vi "Start over Tracking v2.vi"(3 "error in (no error)":errorcluster, 4 "Host System IP Address":string, 5 "VI Path on Host":path) -> (0 "error out":errorcluster, 1 "yes/no?":bool)   [LabVIEW 2016]
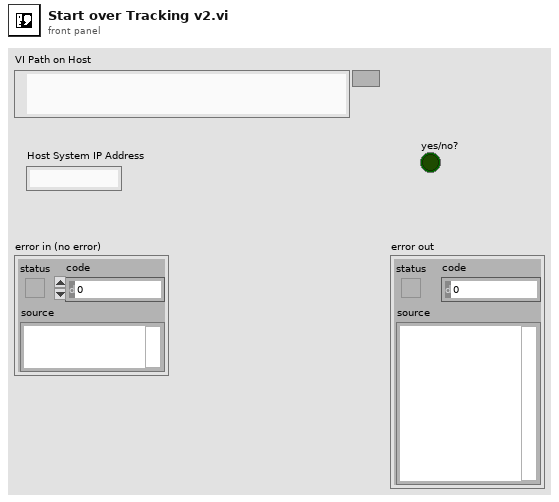
[diagram p1: front panel]
types:
  T1 = enum32{"Invalid", "Standard", "Closed", "Hidden", "Minimized", "Maximized"}
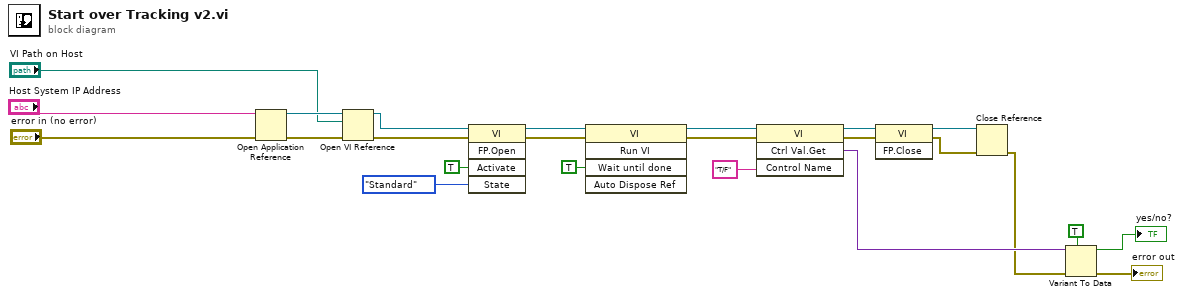
[diagram p0: block diagram]
diagram:
  n1 = Open Application Reference(8:"error in (no error)", 11:"Host System IP Address") -> (0:w9:errorcluster, 3:w10:refnum<vi>)  [unwired: 2 in]
  n2 = Open VI Reference(application reference (local)=w10, vi path="VI Path on Host", error in (no error)=w9) -> (vi reference=w5:refnum<vi>, error out=w6:errorcluster)  [unwired: 3 in]
  n3 = invoke class="VI" method="FP.Open"(reference=w5, error in=w6, "Activate"=TRUE ("Activate?"), "State"=T1."Standard") -> (reference out=w23:refnum<vi>, error out=w22:errorcluster)  [unwired: 1 in, 3 out]
  n4 = invoke class="VI" method="Run VI"(reference=w23, error in=w22, "Wait until done"=TRUE ("Wait Until Done")) -> (reference out=w19:refnum<vi>, error out=w17:errorcluster)  [unwired: 2 in, 3 out]
  n5 = invoke class="VI" method="Ctrl Val.Get"(reference=w19, error in=w17, "Control Name"="T/F") -> (reference out=w12:refnum<vi>, error out=w11:errorcluster, "Get Control Value Variant"=w16:variant)  [unwired: 1 in, 1 out]
  n6 = invoke class="VI" method="FP.Close"(reference=w12, error in=w11) -> (reference out=w3:refnum<vi>, error out=w2:errorcluster)  [unwired: 1 in, 1 out]
  n7 = Close Reference(reference=w3, error in (no error)=w2) -> (error out=w1:errorcluster)
  n8 = Variant To Data(error in=w1, type=TRUE, Variant=w16) -> (data=→"yes/no?":bool, error out=→"error out":errorcluster)
